vi "Configure Reporting.vi"(7 "Custom Reporting Plugin":string, 8 "error in (no error)":errorcluster, 10 "Path":path, 11 "Execution API In":refnum<class "Execution API.lvclass">) -> (0 "error out":errorcluster, 3 "Execution API Out":refnum<class "Execution API.lvclass">)   [LabVIEW 2020, in "Execution API.lvclass"]
doc: "Configure reporting path and toggle automatic report generation.\nIf you have a custom reporting plugin, it can be used by specifying the name of the report class. The report plugin must be installed as defined in LUnit documentation."
uses:
  Execution API.lvclass
  Report Plugin/Report Plugin.lvclass
  C:/git/astemes-lunit/source/Framework/Plugin/Plugin.lvclass
  Execution API.lvclass/Execution API.ctl
  Plugins/XML Report/XML Report.lvclass
  C:/git/astemes-lunit/source/Framework/Report Plugin/Report Plugin.lvclass
  Plugins/Text Report/Text Report.lvclass
  Plugin Loader/Plugin Loader.lvlib
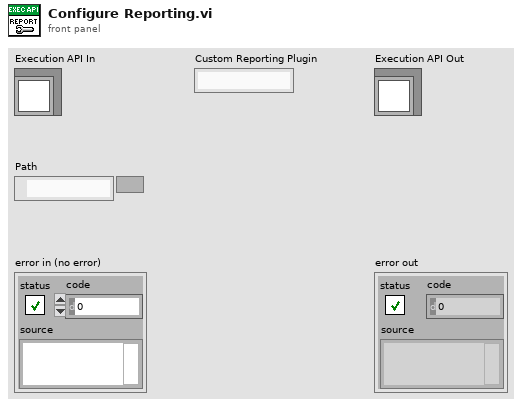
[diagram p1: front panel]
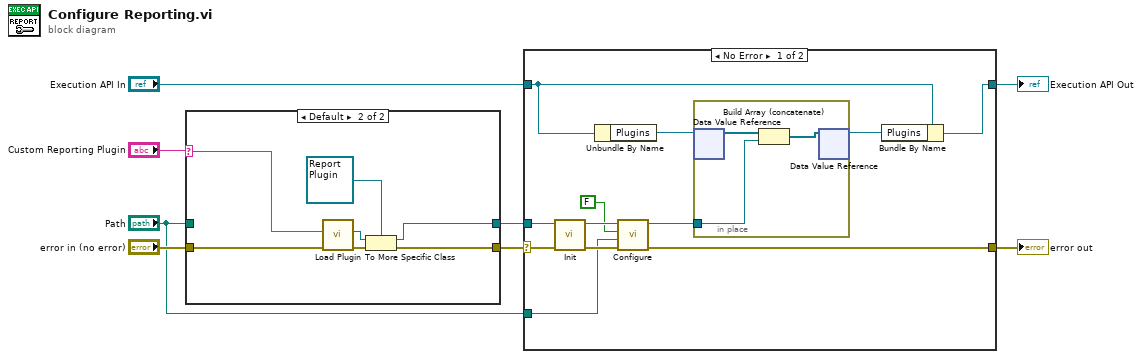
[diagram p0: block diagram]
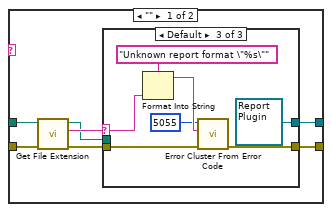
[diagram p2: hidden frame]
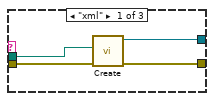
[diagram p3: hidden frame]
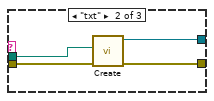
[diagram p4: hidden frame]
diagram:
  n1 = case shown="Default" "Custom Reporting Plugin" {
    selector: "Custom Reporting Plugin" -> [_ w31]
    tunnel: "Path" -> [w15 _]
    tunnel: "error in (no error)" -> [w13 w32]
    tunnel: [w11 w36] -> w3
    tunnel: [w9 w34] -> w4
    frame "" {
      n2 = call <vilib>:"Get File Extension.vi"("error in (no error)"=w13, "file"=w15) -> ("error out"=w12:errorcluster, "lowercase file extension"=w14:string, "dup file"=w10:path)  [unwired: 5 in, 2 out]
      n3 = case shown="Default" w14 {
        selector: w14 -> [_ _ w27]
        tunnel: w12 -> [w19 w23 w30]
        tunnel: [w18 w22 w29] -> w11
        tunnel: w10 -> [w16 w20 _]
        tunnel: [w17 w21 refnum<class "Report Plugin.lvclass"> refnum ("Text Report")] -> w9
        frame "xml" {
          n4 = call "Create.vi"("error in (no error)"=w19, "Report Path"=w16) -> ("error out"=w18:errorcluster, "XML Report"=w17:refnum<class "XML Report.lvclass">)  [unwired: 8 in]
        }
        frame "txt" {
          n5 = call "Create.vi"("error in (no error)"=w23, "Report Path"=w20) -> ("error out"=w22:errorcluster, "Text Report"=w21:refnum<class "Text Report.lvclass">)  [unwired: 8 in]
        }
        frame Default {
          n6 = Format Into String(format string="Unknown report format \"%s\"", w27) -> (resulting string=w26:string)  [unwired: 2 in, 1 out]
          n7 = call <vilib>:"Error Cluster From Error Code.vi"("error in (no error)"=w30, "error message (\"\")"=w26, "error code (0)"=5055) -> ("error out"=w29:errorcluster)  [unwired: 6 in]
        }
      }
    }
    frame Default {
      n8 = call "Load Plugin.vi"("error in (no error)"=w32, "Plugin"=w31) -> ("error out"=w37:errorcluster, "Plugin"=w35:refnum<class "Plugin.lvclass">)  [unwired: 8 in]
      n9 = To More Specific Class(target class=refnum<class "Report Plugin.lvclass"> refnum ("Report Out"), reference=w35, error in=w37) -> (specific class reference=w34:refnum<class "Report Plugin.lvclass">, error out=w36:errorcluster)
    }
  }
  n10 = case shown="No Error" w3 {
    selector: w3 -> [w47 w53]
    tunnel: [w49 w54] -> w6
    tunnel: "Execution API In" -> [w48 w54]
    tunnel: w4 -> [w46 _]
    tunnel: [w43 w53] -> w2
    tunnel: "Path" -> [w42 _]
    frame No Error {
      n11 = call-dynamic "Init.vi"("error in (no error)"=w47, "Plugin in"=w46) -> ("error out"=w44:errorcluster, "Plugin out"=w45:refnum<class "Report Plugin.lvclass">)  [unwired: 8 in]
      n12 = Unbundle By Name(w48) -> ("Plugins"=w39:refnum<data-value>)
      n13 = call-dynamic "Configure.vi"("error in (no error)"=w44, "Path"=w42, "Interactive?"=FALSE, "Report Interface in"=w45) -> ("error out"=w43:errorcluster, "Report Interface out"=w40:refnum<class "Report Plugin.lvclass">)  [unwired: 6 in]
      n14 = in-place {
        in-place-border: w40 -> [w52]
        n15 = in-place-dvr #1(w39) -> (w51:refnum<class "Plugin.lvclass">[])  [unwired: 1 out]
        n16 = Build Array (concatenate)(w51, w52) -> (w50:refnum<class "Plugin.lvclass">[])
        n17 = in-place-dvr #1(w50) -> (w38:refnum<data-value>)  [unwired: 1 out]
      }
      n18 = Bundle By Name(cluster=w48, "Plugins"=w38) -> (w49:refnum<class "Execution API.lvclass">)
    }
    frame Error {
    }
  }
  "error out" <- w2
  "Execution API Out" <- w6
